vi "Raise Error.vi"(7 "message":string, 8 "error in (no error)":errorcluster, 11 "json":string) -> (0 "error out":errorcluster)   [LabVIEW 2019, in "JSON.lvlib"]
doc: "Raises a custom JSON error (code: 538906).\n\nCreated by: Ryan Pacini"
uses:
  JSON.lvlib
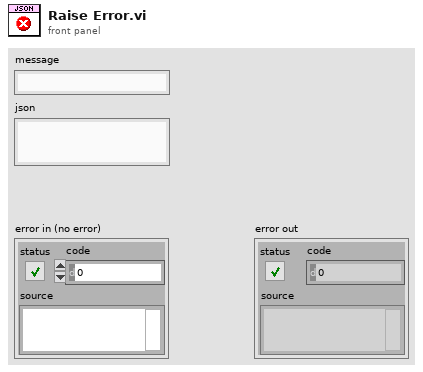
[diagram p1: front panel]
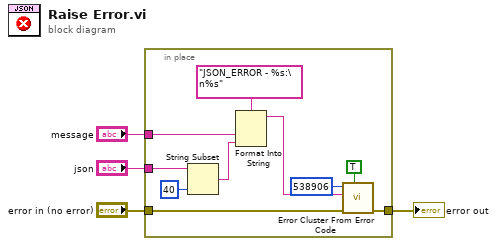
[diagram p0: block diagram]
diagram:
  n1 = in-place {
    in-place-border: "error in (no error)" -> [w14]
    in-place-border: [w13] -> w3
    in-place-border: "json" -> [w12]
    in-place-border: "message" -> [w11]
    n2 = String Subset(string=w12, length (rest)=40 ("length (rest)")) -> (substring=w6:string)  [unwired: 1 in]
    n3 = Format Into String(format string="JSON_ERROR - %s:\n%s", w11, w6) -> (resulting string=w5:string)  [unwired: 2 in, 1 out]
    n4 = call <vilib>:"Error Cluster From Error Code.vi"("show call chain? (False)"=TRUE, "error in (no error)"=w14, "error message (\"\")"=w5, "error code (0)"=538906) -> ("error out"=w13:errorcluster)  [unwired: 5 in]
  }
  "error out" <- w3
